vi "Op-Wait For Trigger Input.vi"(8 "error in (no error)":errorcluster, 9 "timeout (milisec)":i32=5000, 10 "polarity\n(positive:0)":u16(ring) items=["positive", "negative", "either"], 11 "VISA session":refnum<visa-resource-name>) -> (0 "error out":errorcluster, 3 "VISA resource name out":refnum<visa-resource-name>)   [LabVIEW 2016, in "Agilent 415X Series.lvlib"]
doc: "This VI waits for an external trigger at the Extenal Trigger Input BNC connector.\n\nYou can set a timeout value using the TimeOut control to specify how long this VI should wait before return an error, in which case an Instrument Clear will be executed."
uses:
  Agilent 415X Series.lvlib
panel:
  # "* Warning: If TimeOut is set to 0, no timeout will \n  be used by the GPIB wait for RQS VI, as a result,\n  this VI could wait indefinitely for a trigger input."
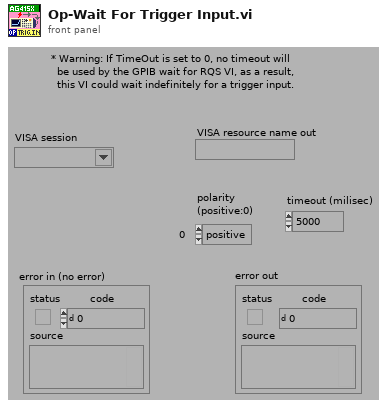
[diagram p1: front panel]
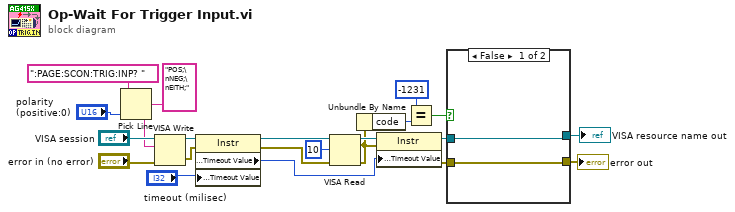
[diagram p0: block diagram]
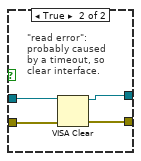
[diagram p2: hidden frame]
diagram:
  n1 = Pick Line(string ("")=":PAGE:SCON:TRIG:INP? ", multi-line string="POS;\nNEG;\nEITH;", line index="polarity\n(positive:0)") -> (output string=w17:string)
  n2 = VISA Write(VISA resource name="VISA session", write buffer=w17, error in (no error)="error in (no error)") -> (VISA resource name out=w11:refnum<visa-resource-name>, error out=w8:errorcluster)  [unwired: 1 out]
  n3 = property class="Instr"(reference=w11, error in=w8, "General Settings:Timeout Value"="timeout (milisec)") -> (reference out=w10:refnum<visa-resource-name>, error out=w9:errorcluster, "General Settings:Timeout Value"=w2:u32)
  n4 = VISA Read(VISA resource name=w10, byte count=u32 10, error in (no error)=w9) -> (VISA resource name out=w4:refnum<visa-resource-name>, error out=w3:errorcluster)  [unwired: 2 out]
  n5 = Unbundle By Name(w3) -> ("code"=w16:i32)
  n6 = property class="Instr"(reference=w4, error in=w3, "General Settings:Timeout Value"=w2) -> (reference out=w6:refnum<visa-resource-name>, error out=w5:errorcluster)
  n7 = Equal?(x=-1231, y=w16) -> (x = y?=w14:bool)
  n8 = case shown="False" w14 {
    tunnel: w6 -> [w23 w28]
    tunnel: w5 -> [w24 w27]
    tunnel: [w24 w26] -> w13
    tunnel: [w23 w25] -> w1
    frame False {
    }
    frame True {
      # "\"read error\":\nprobably caused\nby a timeout, so\nclear interface."
      n9 = VISA Clear(VISA resource name=w28, error in (no error)=w27) -> (VISA resource name out=w25:refnum<visa-resource-name>, error out=w26:errorcluster)
    }
  }
  "error out" <- w13
  "VISA resource name out" <- w1
